vi "OTP-VNA_Extracted_File_Format.vi"(8 "error in (no error)":errorcluster, 9 "Equipment":enum16{"VNA", "LCR"}(ring), 10 "Package Number":string, 11 "File path In (dialog if empty)":path) -> (0 "error out":errorcluster, 2 "Reformatted Ouput":string[][](array[string]), 3 "File path Out (dialog if empty)":path)   [LabVIEW 2020]
uses:
  <vilib>/Utility/file.llb/Read Delimited Spreadsheet (string).vi
  <vilib>/Utility/file.llb/Write Delimited Spreadsheet (string).vi
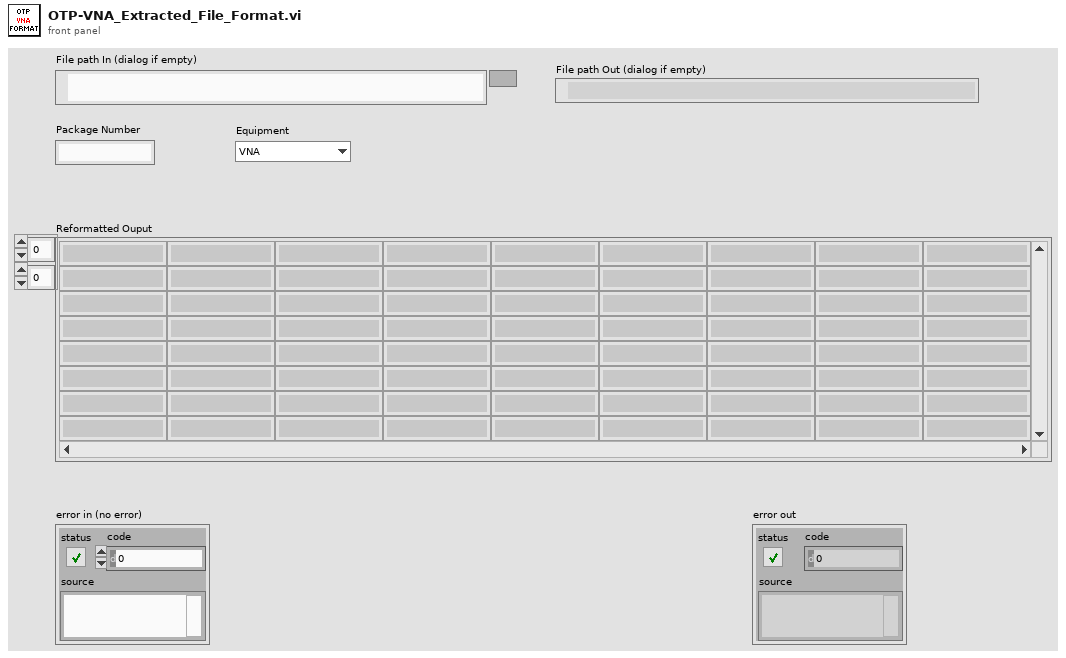
[diagram p1: front panel]
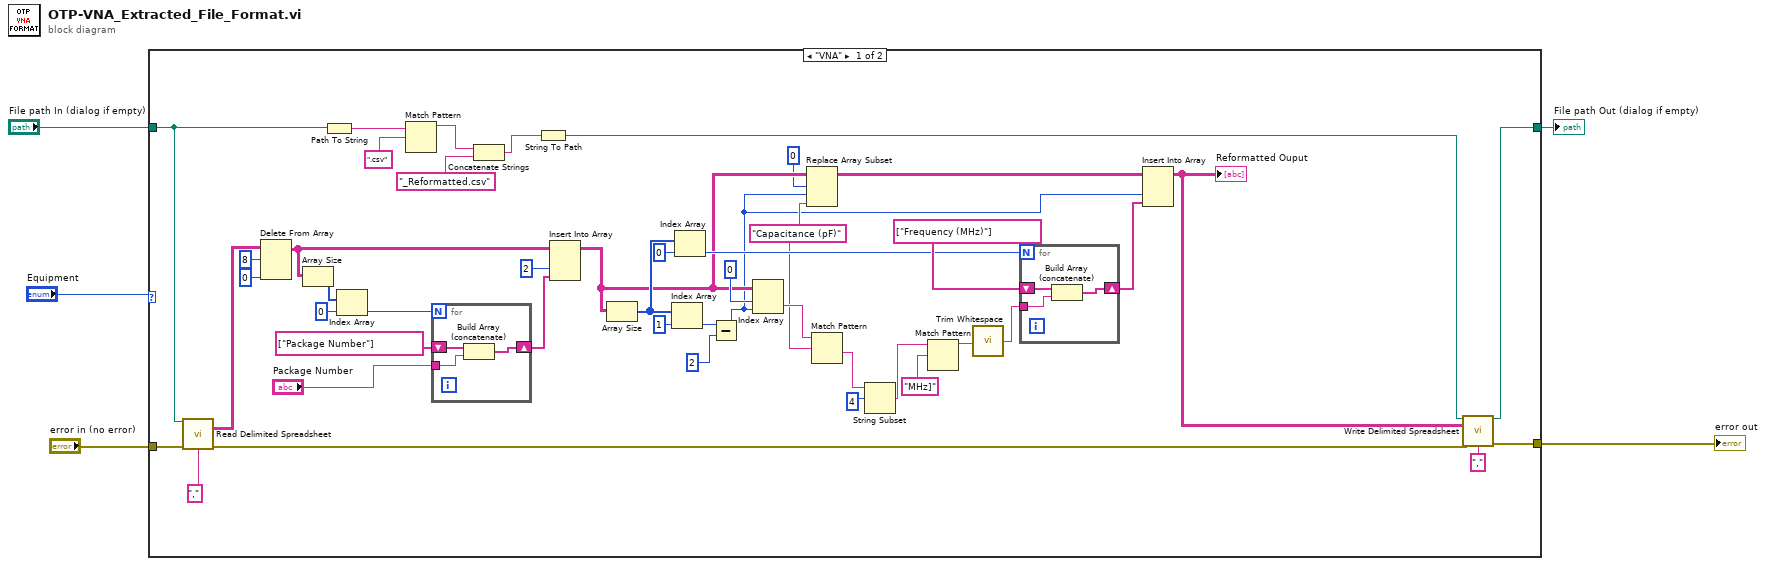
[diagram p0: block diagram]
diagram:
  n1 = case shown="\"VNA\"" "Equipment" {
    tunnel: "File path In (dialog if empty)" -> [w13 w59]
    tunnel: [w51 w58] -> w4
    tunnel: "error in (no error)" -> [w50 w58]
    tunnel: [w6 w59] -> w1
    frame "VNA" {
      w20 = "Capacitance (pF)" ("regular expression")
      n2 = call-poly <vilib>:"Read Delimited Spreadsheet.vi"("file path (dialog if empty)"=w13, "error in (no error)"=w50, "delimiter (\\t)"=",") -> ("all rows"=w49:string[][], "error out"=w14:errorcluster)  [unwired: 7 in, 4 out]
      n3 = Delete From Array(array=w49, length=8, index (row)=0) -> (array with subset deleted=w41:string[][])  [unwired: 1 in, 1 out]
      n4 = Array Size(array=w41) -> (size(s)=w38:i32[])
      n5 = Path To String(path=w13) -> (string=w12:string)
      n6 = Index Array(array=w38, index=0) -> (element=w44:i32)
      n7 = Match Pattern(string=w12, regular expression=".csv") -> (before substring=w10:string)  [unwired: 1 in, 3 out]
      n8 = for {
        N: w44 -> [_]
        shift-right: [w56] -> w39
        shift-left: string[] ["Package Number"] -> [w57]
        tunnel: "Package Number" -> [w55]
        n9 = Build Array (concatenate)(w57, w55) -> (w56:string[])
      }
      n10 = Concatenate Strings(w10, "_Reformatted.csv" ("string")) -> (w8:string)
      n11 = String To Path(string=w8) -> (path=w7:path)
      n12 = Insert Into Array(array=w41, index (col)=2 ("disabled index (col)"), new element=w39) -> (w22:string[][])  [unwired: 1 in]
      n13 = Array Size(array=w22) -> (size(s)=w25:i32[])
      n14 = Index Array(array=w25, index=1) -> (element=w35:i32)
      n15 = Index Array(array=w25, index=0) -> (element=w23:i32)
      n16 = Subtract(x=w35, y=2) -> (x-y=w18:i32)
      n17 = Index Array(array=w22, index (row)=0 ("disabled index (row)"), index (col)=w18) -> (element=w33:string)
      n18 = Replace Array Subset(array=w22, new element=w20, index (row)=0, index (col)=w18) -> (w19:string[][])
      n19 = Match Pattern(string=w33, regular expression=w20) -> (after substring=w32:string)  [unwired: 1 in, 3 out]
      n20 = String Subset(string=w32, offset (0)=4) -> (substring=w30:string)  [unwired: 1 in]
      n21 = Match Pattern(string=w30, regular expression="MHz]") -> (before substring=w28:string)  [unwired: 1 in, 3 out]
      n22 = call <vilib>:"Trim Whitespace.vi"("string"=w28) -> ("trimmed string"=w26:string)  [unwired: 1 in]
      n23 = for {
        N: w23 -> [_]
        shift-right: [w53] -> w17
        shift-left: string[] ["Frequency (MHz)"] -> [w54]
        tunnel: w26 -> [w52]
        n24 = Build Array (concatenate)(w54, w52) -> (w53:string[])
      }
      n25 = Insert Into Array(array=w19, index (col)=w18, new element=w17) -> (w16:string[][])  [unwired: 1 in]
      "Reformatted Ouput" <- w16
      n26 = call-poly <vilib>:"Write Delimited Spreadsheet.vi"("file path (dialog if empty)"=w7, "2D data"=w16, "error in (no error)"=w14, "delimiter (\\t)"="," ("delimiter (\\t)")) -> ("new file path (Not A Path if cancelled)"=w6:path, "error out"=w51:errorcluster)  [unwired: 10 in]
    }
    frame "LCR", Default {
    }
  }
  "error out" <- w4
  "File path Out (dialog if empty)" <- w1
